vi "idd.vi"() -> ()   [LabVIEW 2015]
panel:
  out "hDevice":u32 format="%x"
  in  "idd(szin)":u32[](array[numeric])
  out "idd(szout)":u32[](array[numeric])
  out "idd(out)":u32
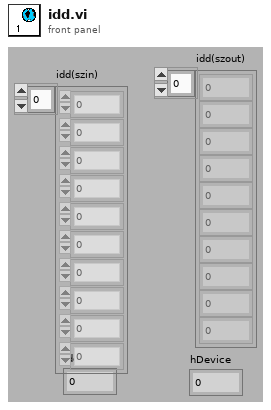
[diagram p1: front panel]
diagram:
